vi "ConvertI16zuU16.vi"(2 "Offset":u16=32768, 4 "file path":path, 5 "Clear string":bool, 6 "BigTiff,Endian":u16(ring)=257 items=["Big-Endian"=0, "Native"=1, "Little-Endian"=2, "BigTiff-Big-Endian"=256, "Bigtiff,Native"=257, "Biftiff,Littleendian"=258]) -> ()   [LabVIEW 2011]
uses:
  TiffModules/ReadTiffPage_I16_text_res.vi
  TiffModules/AddTiffPage_U16_text_res.vi
panel:
  out "Page":i32
  out "string":string
  out "Pixelsize [µm]":cluster{"x":dbl, "y":dbl}
  out "Out":u16[][](graph)
  out "In":i16[][](graph)
  # "will add _U16 to the filename"
  # "works with multi images\nworks with big-TIFF, be sure to select Bigtiff out!\n<32000 and offset 0 for copy"
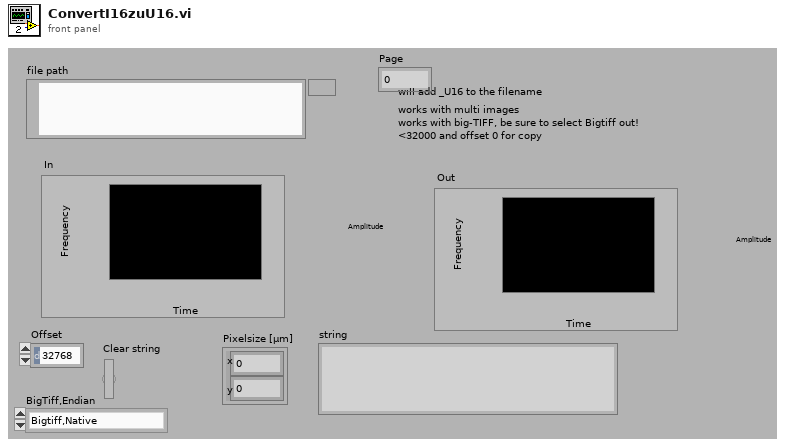
[diagram p1: front panel]
types:
  T1 = cluster{"Tiff refnum":refnum<file>, "BigTiff,Endian":u16}
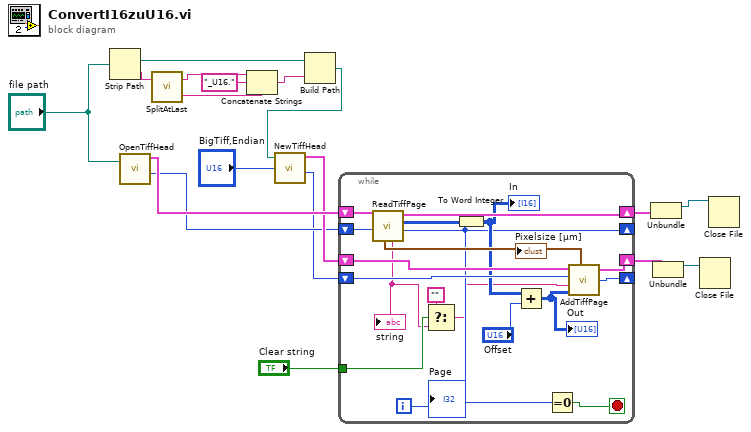
[diagram p0: block diagram]
diagram:
  n1 = Strip Path(path="file path") -> (stripped path=w13:path, name=w18:string)
  n2 = call "OpenTiffHead.vi"("file path"="file path") -> ("TIFF file"=w10:T1, "first Diroffset"=w8:u64)  [unwired: 2 in, 1 out]
  n3 = call "SplitAtLast.vi"("In-String"=w18) -> ("end"=w15:string, "Front (default)"=w17:string)  [unwired: 1 in]
  n4 = Concatenate Strings(w17, "_U16." ("String"), w15) -> (w14:string)
  n5 = Build Path(base path=w13, name or relative path=w14) -> (appended path=w12:path)
  n6 = call "NewTiffHead.vi"("file path"=w12, "BigTiff,Endian"="BigTiff,Endian") -> ("TIFF file"=w9:T1, "Place for first IFD (8,eof-position)"=w7:u64)  [unwired: 2 in, 1 out]
  n7 = while {
    shift-right: [w35] -> w6
    shift-left: w10 -> [w37]
    shift-right: [w34] -> w5
    shift-left: w9 -> [w36]
    shift-right: [w24] -> _
    shift-left: w8 -> [w31]
    shift-right: [w29] -> _
    shift-left: w7 -> [w30]
    tunnel: "Clear string" -> [w22]
    i -> [w23]
    stop <- w25 stop-if-true
    n8 = call-poly "ReadTiffPage.vi"("TIFF file"=w37, "IFDoffset"=w31) -> ("Pixelsize [µm]"=w33:cluster{"x":dbl, "y":dbl}, "TIFF file out"=w35:T1, "16-bit pixmap"=w27:i16[][], "string"=w21:string, "Next offset"=w24:u64)  [unwired: 3 in, 1 out]
    "Pixelsize [µm]" <- w33
    "string" <- w21
    n9 = Select(t="", s=w22, f=w21) -> (s? t:f=w20:string)
    n10 = To Word Integer(number=w27) -> (16bit integer=w26:i16[][])
    "In" <- w26
    n11 = Add(x=w26, y="Offset") -> (x+y=w28:u16[][])
    "Out" <- w28
    n12 = Equal To 0?(x=w24) -> (x = 0?=w25:bool)
    n13 = call-poly "AddTiffPage.vi"("TIFF file"=w36, "After last DIROffset"=w30, "Text"=w20, "16-bit pixmap x, y"=w28, "Pixelsize [µm]"=w33) -> ("TIFF file"=w34:T1, "AfterDIRoffset"=w29:u64)  [unwired: 1 out]
    "Page" <- w23
  }
  n14 = Unbundle(w6) -> ("Tiff refnum"=w4:refnum<file>)  [unwired: 1 out]
  n15 = Unbundle(w5) -> ("Tiff refnum"=w3:refnum<file>)  [unwired: 1 out]
  n16 = Close File(refnum=w3) -> ()  [unwired: 1 in, 2 out]
  n17 = Close File(refnum=w4) -> ()  [unwired: 1 in, 2 out]
